vi "VI_Info_do_Intake_Dashboard.vi"() -> (2 "Sensor_Intake2":dbl, 3 "Sensor_Intake1":dbl, 4 "Intake_State":string)   [LabVIEW 2017]
uses:
  <vilib>/Rock Robotics/Network Tables/NT Read Number.vi
  <vilib>/Rock Robotics/Network Tables/NT Read String.vi
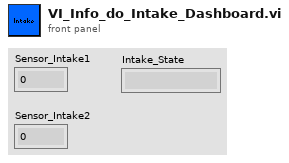
[diagram p1: front panel]
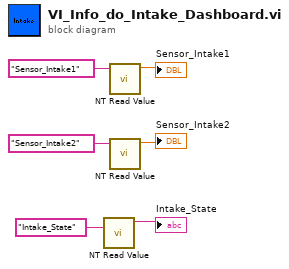
[diagram p0: block diagram]
diagram:
  n1 = call-poly <vilib>:"NT Read Value.vi"("Name"="Intake_State") -> ("String"=→"Intake_State":string)  [unwired: 9 in, 1 out]
  n2 = call-poly <vilib>:"NT Read Value.vi"("Name"="Sensor_Intake1") -> ("Numeric"=→"Sensor_Intake1":dbl)  [unwired: 9 in, 1 out]
  n3 = call-poly <vilib>:"NT Read Value.vi"("Name"="Sensor_Intake2") -> ("Numeric"=→"Sensor_Intake2":dbl)  [unwired: 9 in, 1 out]
